vi "Motor.vi"() -> ()   [LabVIEW 2012]
uses:
  <vilib>/Rock Robotics/SystemInterfaces/DIO/FPGA_DIOPWMChannel.ctl
  <vilib>/Rock Robotics/WPI/MotorControl/WPI_MotorControlOpen Talon.vi
panel:
  in  "Numeric":dbl
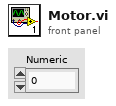
[diagram p1: front panel]
types:
  T1 = typedef "FPGA_DIOPWMChannel.ctl" = enum8{"PWM 1", "PWM 2", "PWM 3", "PWM 4", "PWM 5", "PWM 6", "PWM 7", "PWM 8", "PWM 9", "PWM 10", "Invalid"}
  T2 = typedef "WPI_MotorControlDeviceRef.ctl" = cluster{"DeviceStatus":errorcluster, "Type":enum16{"PWM", "CAN"}, "PWM":cluster{"Digital Module":T3, "PWM Channel":T1, "DeadBand":T4}, "CAN":cluster{"Device Number":u8, "Control Mode":T5, "Semaphore":T6, "Max Vout":dbl}, "Invert":bool, "TransformRef":T7, "InvTransformRef":T7}
  T3 = typedef "FPGA_TypedefDigitalModule.ctl" = enum16{"Digital Module 1", "Digital Module 2"}
  T4 = typedef "WPI_PWMDeadband.ctl" = cluster{"Name":string, "maxPositivePwm":i32, "minPositivePwm":i32, "centerPwm":i32, "maxNegativePwm":i32, "minNegativePwm":i32, "angularRange":u16}
  T5 = typedef "WPI_CANJaguar_ControlMode.ctl" = enum8{"Percent VBus", "Current", "Speed", "Position", "Voltage"}
  T6 = typedef "Semaphore RefNum" = refnum<k1>
  T7 = typedef "WPI_PWMTransform_ConPane.ctl" = refnum<vi>
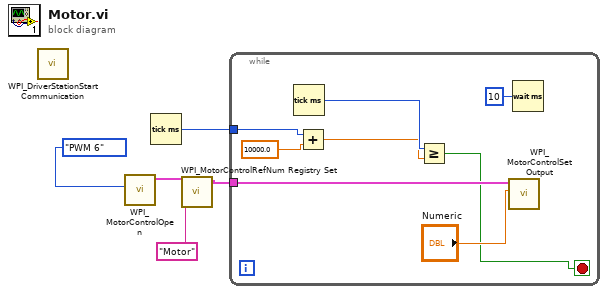
[diagram p0: block diagram]
diagram:
  n1 = call <vilib>:"WPI_DriverStationStart Communication.vi"() -> ()  [unwired: 1 in, 11 out]
  n2 = call-poly <vilib>:"WPI_MotorControlOpen.vi"("PWM Channel"=FPGA_DIOPWMChannel."PWM 6") -> ("MotorControlDeviceRef"=w4:T2)  [unwired: 9 in, 1 out]
  n3 = Tick Count (ms)() -> (millisecond timer value=w1:u32)
  n4 = call <vilib>:"WPI_MotorControlRefNum Registry Set.vi"("refnum name"="Motor", "MotorControlDevRef"=w4) -> ("MotorControlDevRef"=w3:T2)  [unwired: 8 in, 1 out]
  n5 = while {
    tunnel: w3 -> [w13]
    tunnel: w1 -> [w7]
    stop <- w9 stop-if-true
    n6 = Tick Count (ms)() -> (millisecond timer value=w10:u32)
    n7 = Add(x=w7, y=10000.0) -> (x+y=w6:dbl)
    n8 = Greater Or Equal?(x=w10, y=w6) -> (x >= y?=w9:bool)
    n9 = call <vilib>:"WPI_MotorControlSetOutput.vi"("Output"="Numeric", "MotorControlDevRef"=w13) -> ()  [unwired: 7 in, 3 out]
    n10 = Wait (ms)(milliseconds to wait=u32 10) -> ()  [unwired: 1 out]
  }
